vi "RecvOneBmuVolt _Show.vi"(0 "BMU NO":i32=10, 1 "类型":u32(ring)=4 items=["PCI5121"=1, "PCI9810"=2, "USBCAN1"=3, "USBCAN2"=4, "PCI9820"=5, "CAN232"=6, "PCI5110"=7, "CANLite(mini)"=8, "ISA9620"=9, "ISA5420"=10, "PC104CAN"=11, "CANET"=17, "DNP9810"=13, "USBCAN-E-U"=20, "USBCAN-2E-U"=21], 2 "设备索引":u32(ring) items=["0", "1", "2", "3", "4", "5", "6", "7", "8", "9", "10", "11", "12", "13", "14", "15", ""], 3 "CAN路数":u32(ring) items=["0", "1"], 5 "MyIndex":dbl, 11 "time out":u32, 12 "VoltNumber":u64, 13 "Range_MinVolt":dbl, 14 "NtcNumber":u64, 15 "MinTempLimit":dbl) -> (4 "Volt":dbl[](array[numeric]), 6 "Horizontal":i16, 8 "Vertical":i16, 10 "温度temp":dbl[](array[numeric]))   [LabVIEW 2013]
panel:
  out "x < y?":bool
  out "温度":T1
  in  "错误输入":errorcluster
  out "Time":dbl
  in  "Range_MinVolt 2":dbl
  out "电压":T2
  # "BMU单体采集"
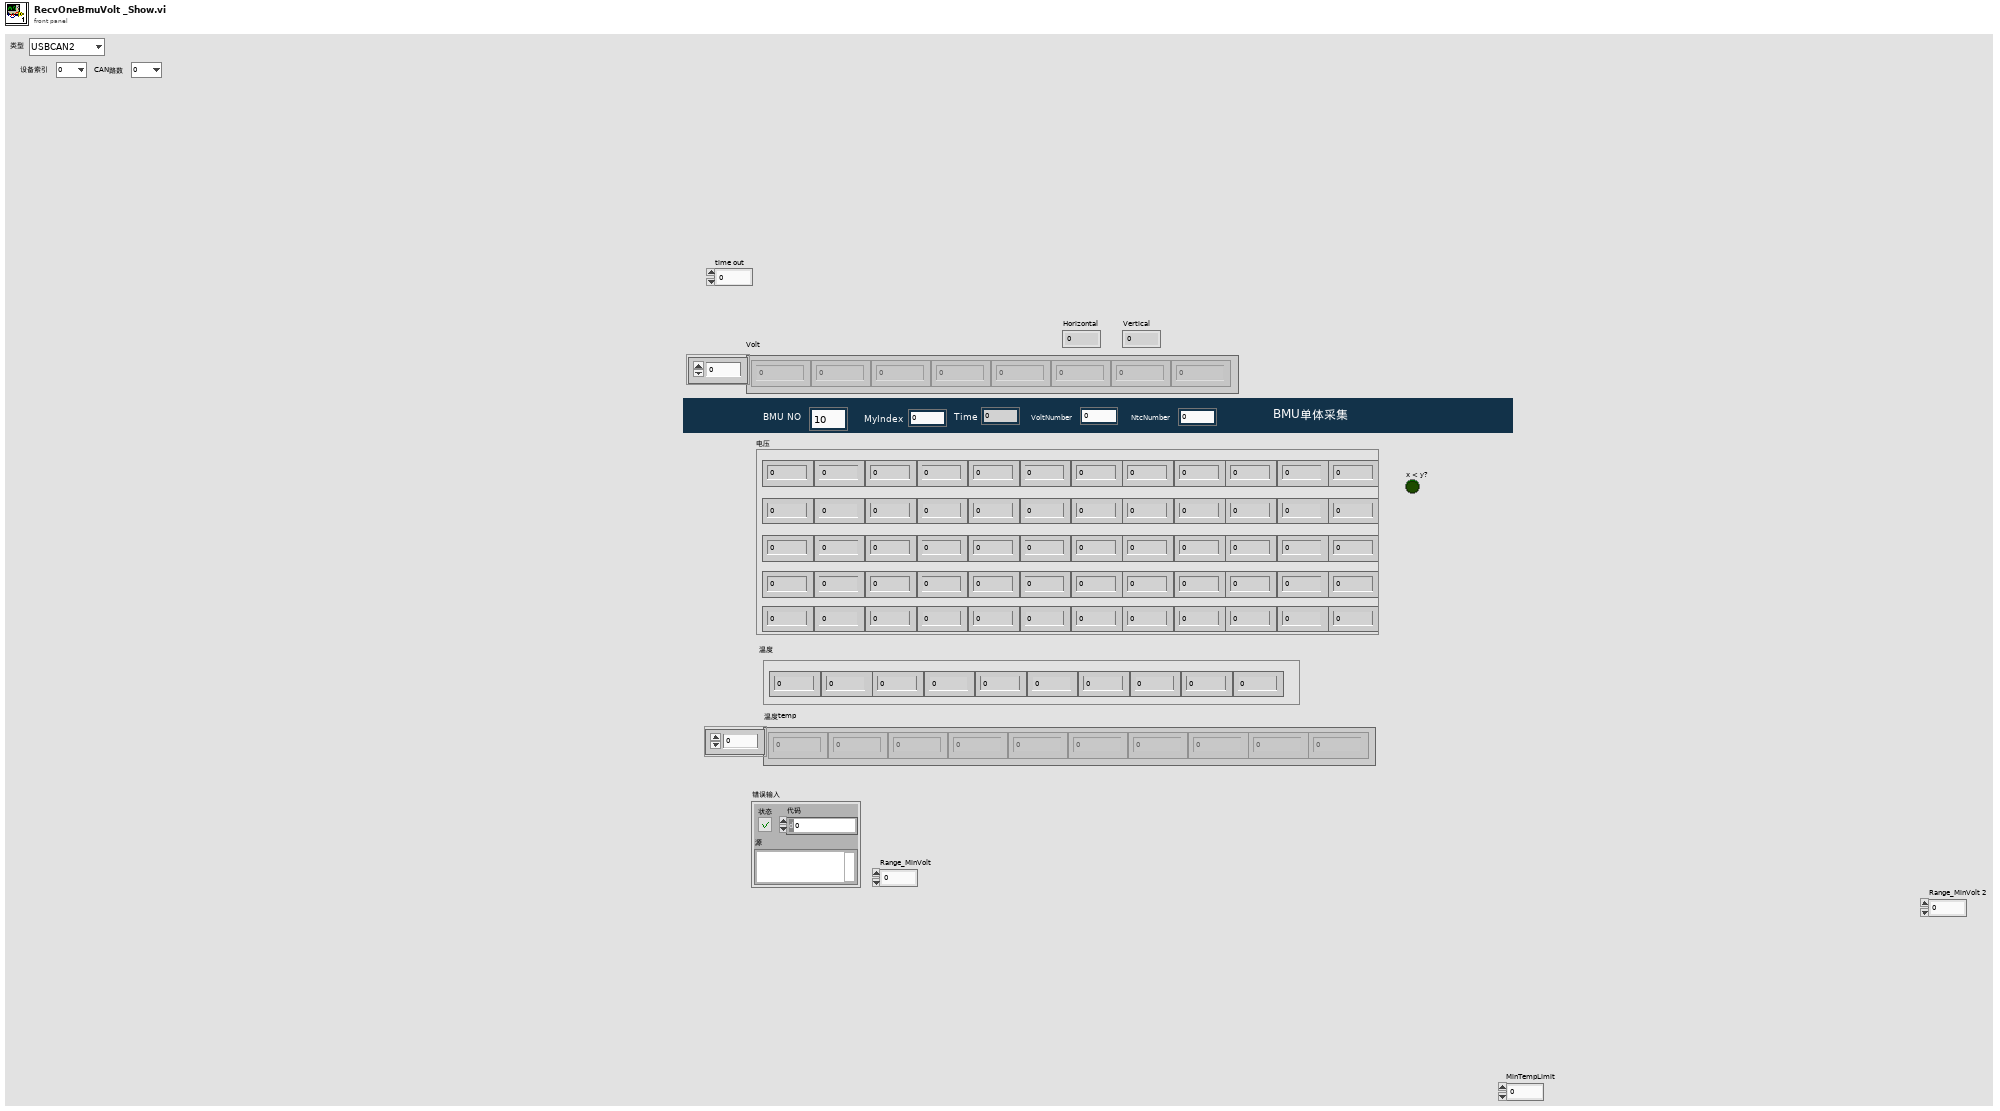
[diagram p1: front panel]
types:
  T1 = cluster{"数值输入控件":dbl, "数值输入控件 2":dbl, "数值输入控件 3":dbl, "数值输入控件 4":dbl, "数值输入控件 5":dbl, "数值输入控件 6":dbl, "数值输入控件 7":dbl, "数值输入控件 8":dbl, "数值输入控件 9":dbl, "数值输入控件 10":dbl}
  T2 = cluster{"数值输入控件":dbl, "数值输入控件 2":dbl, "数值输入控件 3":dbl, "数值输入控件 4":dbl, "数值输入控件 5":dbl, "数值输入控件 6":dbl, "数值输入控件 7":dbl, "数值输入控件 8":dbl, "数值输入控件 9":dbl, "数值输入控件 10":dbl, "数值输入控件 11":dbl, "数值输入控件 12":dbl, "数值输入控件 13":dbl, "数值输入控件 14":dbl, "数值输入控件 15":dbl, "数值输入控件 16":dbl, "数值输入控件 17":dbl, "数值输入控件 18":dbl, "数值输入控件 19":dbl, "数值输入控件 20":dbl, "数值输入控件 21":dbl, "数值输入控件 22":dbl, "数值输入控件 23":dbl, "数值输入控件 24":dbl, "数值输入控件 25":dbl, "数值输入控件 26":dbl, "数值输入控件 27":dbl, "数值输入控件 28":dbl, "数值输入控件 29":dbl, "数值输入控件 30":dbl, "数值输入控件 31":dbl, "数值输入控件 32":dbl, "数值输入控件 33":dbl, "数值输入控件 34":dbl, "数值输入控件 35":dbl, "数值输入控件 36":dbl, "数值输入控件 37":dbl, "数值输入控件 38":dbl, "数值输入控件 39":dbl, "数值输入控件 40":dbl, "数值输入控件 41":dbl, "数值输入控件 42":dbl, "数值输入控件 43":dbl, "数值输入控件 44":dbl, "数值输入控件 45":dbl, "数值输入控件 46":dbl, "数值输入控件 47":dbl, "数值输入控件 48":dbl, "数值输入控件 49":dbl, "数值输入控件 50":dbl, "数值输入控件 51":dbl, "数值输入控件 52":dbl, "数值输入控件 53":dbl, "数值输入控件 54":dbl, "数值输入控件 55":dbl, "数值输入控件 56":dbl, "数值输入控件 57":dbl, "数值输入控件 58":dbl, "数值输入控件 59":dbl, "数值输入控件 60":dbl}
  T3 = cluster{"Volt[0]":dbl, "Volt[1]":dbl, "Volt[2]":dbl, "Volt[3]":dbl, "Volt[4]":dbl, "Volt[5]":dbl, "Volt[6]":dbl, "Volt[7]":dbl, "Volt[8]":dbl, "Volt[9]":dbl, "Volt[10]":dbl, "Volt[11]":dbl, "Volt[12]":dbl, "Volt[13]":dbl, "Volt[14]":dbl, "Volt[15]":dbl, "Volt[16]":dbl, "Volt[17]":dbl, "Volt[18]":dbl, "Volt[19]":dbl, "Volt[20]":dbl, "Volt[21]":dbl, "Volt[22]":dbl, "Volt[23]":dbl, "Volt[24]":dbl, "Volt[25]":dbl, "Volt[26]":dbl, "Volt[27]":dbl, "Volt[28]":dbl, "Volt[29]":dbl, "Volt[30]":dbl, "Volt[31]":dbl, "Volt[32]":dbl, "Volt[33]":dbl, "Volt[34]":dbl, "Volt[35]":dbl, "Volt[36]":dbl, "Volt[37]":dbl, "Volt[38]":dbl, "Volt[39]":dbl, "Volt[40]":dbl, "Volt[41]":dbl, "Volt[42]":dbl, "Volt[43]":dbl, "Volt[44]":dbl, "Volt[45]":dbl, "Volt[46]":dbl, "Volt[47]":dbl, "Volt[48]":dbl, "Volt[49]":dbl, "Volt[50]":dbl, "Volt[51]":dbl, "Volt[52]":dbl, "Volt[53]":dbl, "Volt[54]":dbl, "Volt[55]":dbl, "Volt[56]":dbl, "Volt[57]":dbl, "Volt[58]":dbl, "Volt[59]":dbl}
  T4 = cluster{"ID":u32, "TimeStamp":u32, "TimeFlag":u8, "SendType":u8, "RemoteFlag":u8, "ExternFlag":u8, "DataLen":u8, u8, u8, u8, u8, u8, u8, u8, u8, u8, u8, u8}
  T5 = cluster{"温度temp[0]":dbl, "温度temp[1]":dbl, "温度temp[2]":dbl, "温度temp[3]":dbl, "温度temp[4]":dbl, "温度temp[5]":dbl, "温度temp[6]":dbl, "温度temp[7]":dbl, "温度temp[8]":dbl, "温度temp[9]":dbl}
  T6 = typedef "LVPointTypeDef.ctl" = cluster{"Horizontal":i16, "Vertical":i16}
  T7 = typedef "LVRectTypeDef.ctl" = cluster{"Left":i16, "Top":i16, "Right":i16, "Bottom":i16}
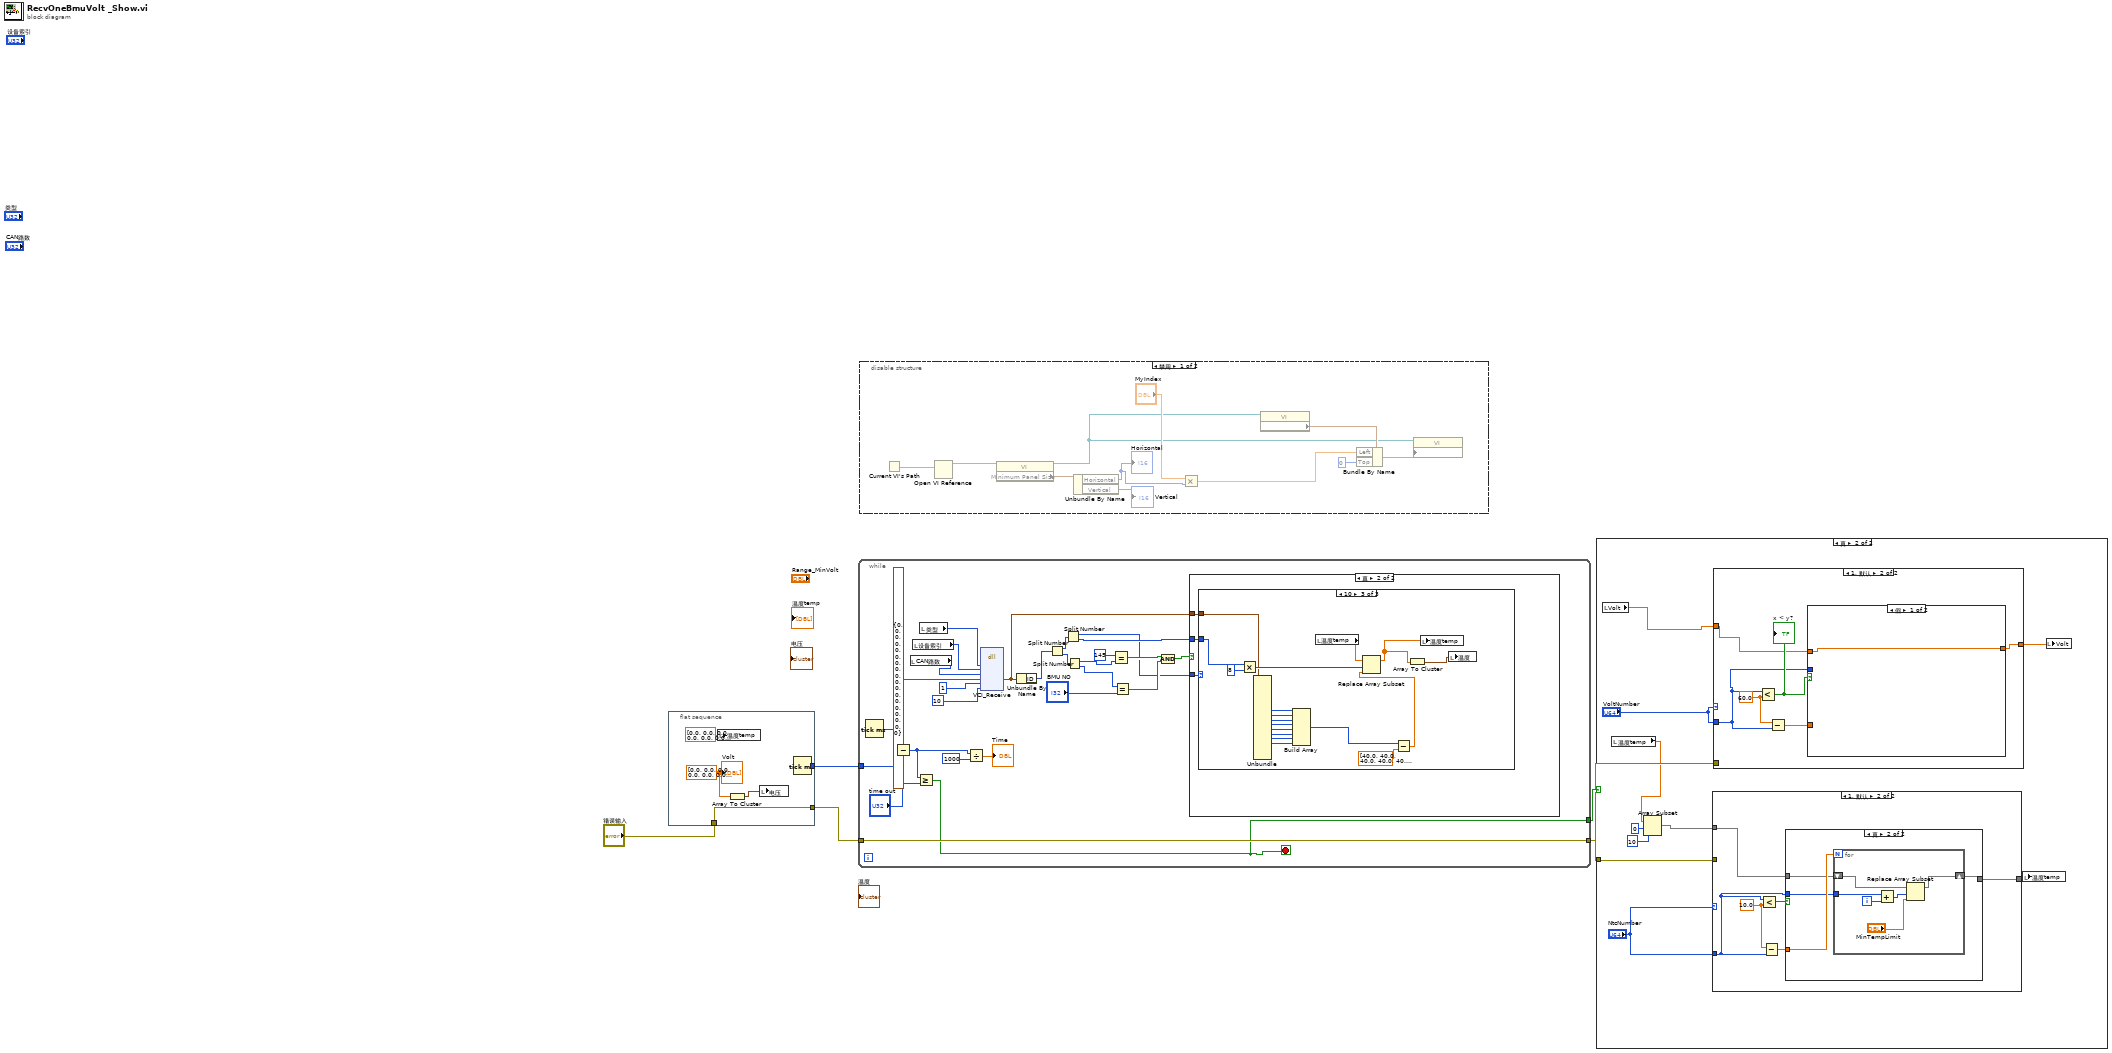
[diagram p0: block diagram]
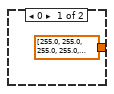
[diagram p3: hidden frame]
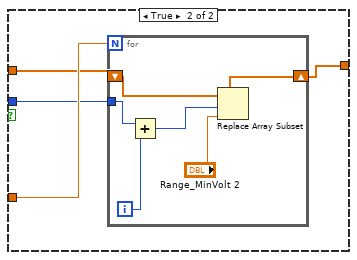
[diagram p4: hidden frame]
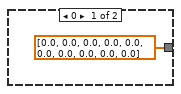
[diagram p5: hidden frame]
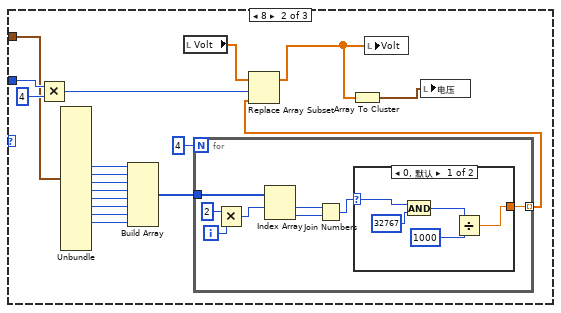
[diagram p10: hidden frame]
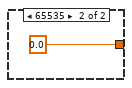
[diagram p11: hidden frame]
diagram:
  n1 = flat-sequence {
    tunnel: [w10] -> w5
    tunnel: [w6] -> w3
    tunnel: "错误输入" -> [w6]
    frame #0 {
      w9 = dbl[] [0.0, 0.0, 0.0, 0.0, 0.0, 0.0, 0.0, 0.0, 0.0, 0.0, 0.0, 0.0, 0.0, 0.0, 0.0, 0.0, 0.0, 0.0, 0.0, 0.0, 0.0, 0.0, 0.0, 0.0, 0.0, 0.0, 0.0, 0.0, 0.0, 0.0, 0.0, 0.0, 0.0, 0.0, 0.0, 0.0, 0.0, 0.0, 0.0, 0.0, 0.0, 0.0, 0.0, 0.0, 0.0, 0.0, 0.0, 0.0, 0.0, 0.0, 0.0, 0.0, 0.0, 0.0, 0.0, 0.0, 0.0, 0.0, 0.0, 0.0] ("Volt")
      n2 = local write "温度temp"(dbl[] [0.0, 0.0, 0.0, 0.0, 0.0, 0.0, 0.0, 0.0, 0.0, 0.0] ("温度mp")) -> ()
      n3 = Array To Cluster(array=w9) -> (cluster=w8:T3)
      n4 = local write "电压"(w8) -> ()
      n5 = Tick Count (ms)() -> (millisecond timer value=w10:u32)
      "Volt" <- w9
    }
  }
  n6 = while {
    tunnel: w5 -> [w30]
    tunnel: [w12] -> w4
    tunnel: w3 -> [w12]
    tunnel: [w11] -> w1
    stop <- w11 stop-if-true
    n7 = Tick Count (ms)() -> (millisecond timer value=w31:u32)
    n8 = Subtract(x=w31, y=w30) -> (x-y=w16:u32)
    n9 = local read "CAN路数"() -> (w35:u32)
    n10 = local read "设备索引"() -> (w32:u32)
    n11 = Greater Or Equal?(x=w16, y="time out") -> (x >= y?=w11:bool)
    n12 = local read "类型"() -> (w33:u32)
    n13 = Divide(x=w16, y=u32 1000) -> (x/y=→"Time":dbl)
    n14 = dll-call lib="PTH1rabs FBluewave New EnergySVN_Work二代自动化AutoBurn - dll - Don't Init CanSettingsControlCAN.dll" fn="VCI_Receive"("DeviceType"=w33, "DeviceInd"=w32, "CANInd"=w35, "pReceive"=T4 {"ID"=0, "TimeStamp"=0, "TimeFlag"=0, "SendType"=0, "RemoteFlag"=0, "ExternFlag"=0, "DataLen"=0, 0, 0, 0, 0, 0, 0, 0, 0, 0, 0, 0}, "Len"=u32 1, "WaitTime"=10) -> ("pReceive"=w18:T4)  [unwired: 8 in, 3 out]
    n15 = Unbundle By Name(w18) -> ("ID"=w28:u32)
    n16 = Split Number(x=w28) -> (hi(x)=w27:u16, lo(x)=w26:u16)
    n17 = Split Number(x=w27) -> (hi(x)=w13:u8, lo(x)=w17:u8)
    n18 = Split Number(x=w26) -> (hi(x)=w24:u8, lo(x)=w23:u8)
    n19 = Equal?(x=u8 145, y=w24) -> (x = y?=w21:bool)
    n20 = Equal?(x=w23, y="BMU NO") -> (x = y?=w20:bool)
    n21 = Compound Arithmetic op=AND(w21, w20) -> (w19:bool)
    n22 = case shown="真" w19 {
      tunnel: w18 -> [_ w39]
      tunnel: w17 -> [_ w40]
      tunnel: w13 -> [_ w38]
      frame False {
      }
      frame True {
        n23 = case shown="10" w38 {
          tunnel: w40 -> [_ w57 w76]
          tunnel: w39 -> [_ w54 w74]
          frame 0, Default {
          }
          frame 8 {
            n24 = Multiply(x=w57, y=u8 4) -> (x*y=w55:u8)
            n25 = Unbundle(w54) -> (w53:u8, w52:u8, w51:u8, w50:u8, w49:u8, w48:u8, w47:u8, w46:u8)  [unwired: 10 out]
            n26 = Build Array(w53, w52, w51, w50, w49, w48, w47, w46) -> (w45:u8[])
            n27 = local read "Volt"() -> (w58:dbl[])
            n28 = for {
              N: 4 -> [_]
              tunnel: w45 -> [w66]
              tunnel: [w59] -> w44 mode=indexing
              i -> [w65]
              n29 = Multiply(x=2, y=w65) -> (x*y=w63:i32)
              n30 = Index Array(array=w66, index #1=w63) -> (element #1=w62:u8, element #2=w61:u8)  [unwired: 1 in]
              n31 = Join Numbers(hi=w62, lo=w61) -> ((hi.lo)=w60:u16)
              n32 = case shown="0, 默认" w60 {
                selector: w60 -> [w71 _]
                tunnel: [w67 0.0 ("数值输入控件")] -> w59
                frame 0, Default {
                  n33 = And(x=w71, y=u16 32767) -> (x .and. y?=w69:u16)
                  n34 = Divide(x=w69, y=u16 1000) -> (x/y=w67:dbl)
                }
                frame 65535 {
                }
              }
            }
            n35 = Replace Array Subset(array=w58, new element=w44, index=w55) -> (w41:dbl[])
            n36 = Array To Cluster(array=w41) -> (cluster=w42:T3)
            n37 = local write "Volt"(w41) -> ()
            n38 = local write "电压"(w42) -> ()
          }
          frame 16 {
            n39 = Multiply(x=w76, y=u8 8) -> (x*y=w79:u8)
            n40 = Unbundle(w74) -> (w80:u8, w81:u8, w82:u8, w83:u8, w84:u8, w85:u8, w86:u8, w87:u8)  [unwired: 10 out]
            n41 = Build Array(w80, w81, w82, w83, w84, w85, w86, w87) -> (w88:u8[])
            n42 = local read "温度temp"() -> (w77:dbl[])
            n43 = Subtract(x=w88, y=dbl[] [40.0, 40.0, 40.0, 40.0, 40.0, 40.0, 40.0, 40.0, 40.0, 40.0, 40.0, 40.0, 40.0, 40.0, 40.0, 40.0]) -> (x-y=w90:dbl[])
            n44 = Replace Array Subset(array=w77, new element=w90, index=w79) -> (w73:dbl[])
            n45 = Array To Cluster(array=w73) -> (cluster=w75:T5)
            n46 = local write "温度temp"(w73) -> ()
            n47 = local write "温度"(w75) -> ()
          }
        }
      }
    }
  }
  n48 = disable-structure shown="禁用" {
    frame Disabled {
      n49 = Current VI's Path() -> (path=w101:path)
      n50 = Open VI Reference(vi path=w101) -> (vi reference=w100:refnum<vi>)  [unwired: 5 in, 1 out]
      n51 = property class="VI"(reference=w100) -> (reference out=w91:refnum<vi>, "Minimum Panel Size"=w98:T6)  [unwired: 1 in, 1 out]
      n52 = Unbundle By Name(w98) -> ("Horizontal"=w96:i16, "Vertical"=→"Vertical":i16)
      "Horizontal" <- w96
      n53 = Multiply(x="MyIndex", y=w96) -> (x*y=w92:dbl)
      n54 = property class="VI"(reference=w91) -> ("Front Panel.WinBounds"=w94:T7)  [unwired: 1 in, 2 out]
      n55 = Bundle By Name(cluster=w94, "Left"=w92, "Top"=i16 0) -> (w95:T7)
      n56 = property class="VI"(reference=w91, "Front Panel.WinBounds"=w95) -> ()  [unwired: 1 in, 2 out]
    }
    frame Enabled {
    }
  }
  n57 = case shown="真" w1 {
    tunnel: w4 -> [_ w106]
    frame False {
    }
    frame True {
      n58 = local read "Volt"() -> (w104:dbl[])
      n59 = local read "温度temp"() -> (w103:dbl[])
      n60 = Array Subset(array=w103, index=0 ("索引"), length=10 ("长度")) -> (w108:dbl[])
      n61 = case shown="1, 默认" "NtcNumber" {
        tunnel: w108 -> [_ w133]
        tunnel: [dbl[] [0.0, 0.0, 0.0, 0.0, 0.0, 0.0, 0.0, 0.0, 0.0, 0.0] w132] -> w105
        tunnel: "NtcNumber" -> [_ w131]
        tunnel: w106 -> [_ _]
        frame 0 {
        }
        frame 1, Default {
          w135 = 10.0 ("y")
          n62 = Less?(x=w131, y=w135) -> (x < y?=w136:bool)
          n63 = Subtract(x=w135, y=w131) -> (x-y=w134:dbl)
          n64 = case shown="真" w136 {
            tunnel: w133 -> [w137 w140]
            tunnel: [w137 w138] -> w132
            tunnel: w134 -> [_ w141]
            tunnel: w131 -> [_ w139]
            frame False {
            }
            frame True {
              n65 = for {
                N: w141 -> [_]
                shift-right: [w146] -> w138
                shift-left: w140 -> [w147]
                tunnel: w139 -> [w145]
                i -> [w144]
                n66 = Add(x=w145, y=w144) -> (x+y=w143:u64)
                n67 = Replace Array Subset(array=w147, new element="MinTempLimit", index=w143) -> (w146:dbl[])
              }
            }
          }
        }
      }
      n68 = case shown="1, 默认" "VoltNumber" {
        tunnel: "VoltNumber" -> [_ w115]
        tunnel: [dbl[] [255.0, 255.0, 255.0, 255.0, 255.0, 255.0, 255.0, 255.0, 255.0, 255.0, 255.0, 255.0, 255.0, 255.0, 255.0, 255.0, 255.0, 255.0, 255.0, 255.0, 255.0, 255.0, 255.0, 255.0, 255.0, 255.0, 255.0, 255.0, 255.0, 255.0, 255.0, 255.0, 255.0, 255.0, 255.0, 255.0, 255.0, 255.0, 255.0, 255.0, 255.0, 255.0, 255.0, 255.0, 255.0, 255.0, 255.0, 255.0, 255.0, 255.0, 255.0, 255.0, 255.0, 255.0, 255.0, 255.0, 255.0, 255.0, 255.0, 255.0] ("电压") w114] -> w102
        tunnel: w104 -> [_ w113]
        tunnel: w106 -> [_ _]
        frame 0 {
        }
        frame 1, Default {
          w117 = 60.0 ("y")
          n69 = Less?(x=w115, y=w117) -> (x < y?=w118:bool)
          "x < y?" <- w118
          n70 = Subtract(x=w117, y=w115) -> (x-y=w116:dbl)
          n71 = case shown="假" w118 {
            tunnel: w113 -> [w119 w122]
            tunnel: [w119 w120] -> w114
            tunnel: w116 -> [_ w123]
            tunnel: w115 -> [_ w121]
            frame False {
            }
            frame True {
              n72 = for {
                N: w123 -> [_]
                shift-right: [w128] -> w120
                shift-left: w122 -> [w129]
                tunnel: w121 -> [w127]
                i -> [w126]
                n73 = Add(x=w127, y=w126) -> (x+y=w125:u64)
                n74 = Replace Array Subset(array=w129, new element="Range_MinVolt 2", index=w125) -> (w128:dbl[])
              }
            }
          }
        }
      }
      n75 = local write "温度temp"(w105) -> ()
      n76 = local write "Volt"(w102) -> ()
    }
  }
